vi "Get Visible Chart Data.vi"(7 "Selection Chart":refnum<vi>, 9 "error in (no error)":errorcluster) -> (1 "error out":errorcluster, 2 "waveform out":waveform(dbl), 4 "Y Length":i32)   [LabVIEW 2012]
uses:
  <vilib>/Waveform/WDTOps.llb/WDT Append Waveforms DBL.vi
  <vilib>/Waveform/WDTOps.llb/WDT Get Waveform Subset DBL.vi
panel:
  out "Time":dbl
  out "Portion":dbl
  out "size(s)":i32
  out "t0":timestamp
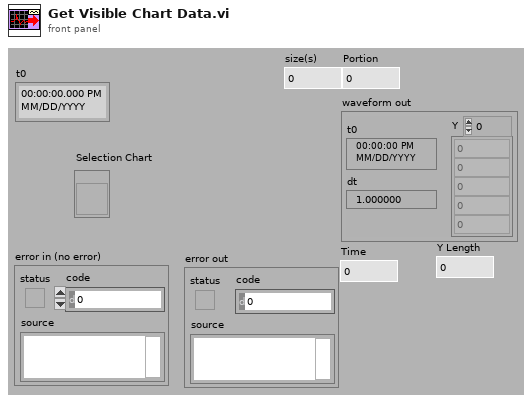
[diagram p1: front panel]
types:
  T1 = typedef "LVRangeTypeDef.ctl" = cluster{"Minimum":dbl, "Maximum":dbl, "Increment":dbl, "Minor Increment":dbl, "Start":dbl}
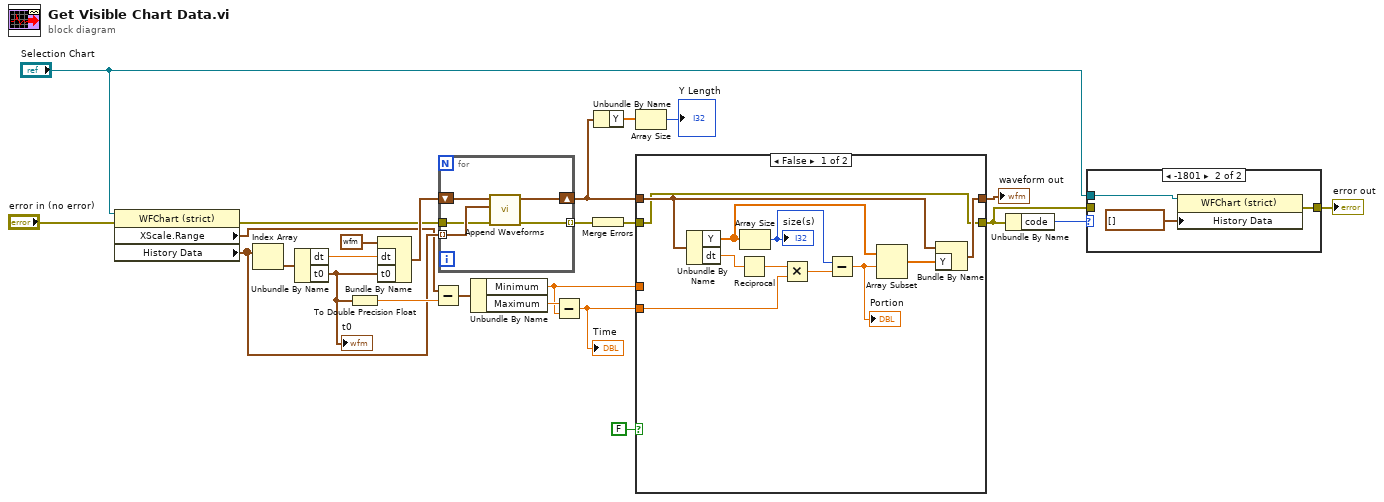
[diagram p0: block diagram]
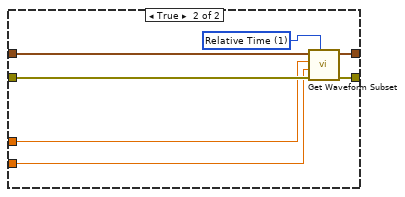
[diagram p2: hidden frame]
diagram:
  n1 = property class="WFChart (strict)"(reference="Selection Chart", error in="error in (no error)") -> (error out=w18:errorcluster, "XScale.Range"=w3:T1, "History Data"=w7:waveform(dbl)[])  [unwired: 1 out]
  n2 = Index Array(array=w7) -> (element=w6:waveform(dbl))  [unwired: 1 in]
  n3 = Unbundle By Name(w6) -> ("dt"=w20:dbl, "t0"=w17:timestamp)
  "t0" <- w17
  n4 = To Double Precision Float(number=w17) -> (double precision float=w15:dbl)
  n5 = Bundle By Name(cluster=waveform(dbl) {"t0"=timestamp(0 s since 1904-01-01), "dt"=2.267573696145e-05, "Y"=[]} ("waveform out"), "dt"=w20, "t0"=w17) -> (w22:waveform(dbl))
  n6 = Subtract(x=w3, y=w15) -> (x-y=w16:T1)
  n7 = for {
    tunnel: w7 -> [w29] mode=indexing
    shift-right: [w30] -> w5
    shift-left: w22 -> [w28]
    tunnel: w18 -> [w27]
    tunnel: [w26] -> w23 mode=indexing
    n8 = call-poly <vilib>:"Append Waveforms.vi"("error in (no error)"=w27, "waveform B"=w29, "waveform A"=w28) -> ("error out"=w26:errorcluster, "waveform out"=w30:waveform(dbl))  [unwired: 7 in]
  }
  n9 = Unbundle By Name(w16) -> ("Minimum"=w4:dbl, "Maximum"=w21:dbl)
  n10 = Subtract(x=w21, y=w4) -> (x-y=w2:dbl)
  "Time" <- w2
  n11 = Merge Errors(w23) -> (w24:errorcluster)
  n12 = Unbundle By Name(w5) -> ("Y"=w9:dbl[])
  n13 = Array Size(array=w9) -> (size(s)=→"Y Length":i32)
  n14 = case shown="False" FALSE {
    tunnel: w24 -> [w31 w48]
    tunnel: [w31 w46] -> w12
    tunnel: [w32 w45] -> w10
    tunnel: w5 -> [w35 w44]
    tunnel: w4 -> [_ w43]
    tunnel: w2 -> [w40 w42]
    frame False {
      n15 = Unbundle By Name(w35) -> ("Y"=w36:dbl[], "dt"=w38:dbl)
      n16 = Reciprocal(x=w38) -> (1/x=w37:dbl)
      n17 = Array Size(array=w36) -> (size(s)=w41:i32)
      "size(s)" <- w41
      n18 = Multiply(x=w37, y=w40) -> (x*y=w39:dbl)
      n19 = Subtract(x=w41, y=w39) -> (x-y=w33:dbl)
      "Portion" <- w33
      n20 = Array Subset(array=w36, index=w33) -> (w34:dbl[])  [unwired: 1 in]
      n21 = Bundle By Name(cluster=w35, "Y"=w34) -> (w32:waveform(dbl))
    }
    frame True {
      w47 = u16 1 items=["Samples", "Relative Time"] ("start/duration format")
      n22 = call-poly <vilib>:"Get Waveform Subset.vi"("start/duration format"=w47, "error in (no error)"=w48, "duration"=w42, "start samples/time"=w43, "waveform in"=w44) -> ("error out"=w46:errorcluster, "waveform out"=w45:waveform(dbl))  [unwired: 1 in, 2 out]
    }
  }
  "waveform out" <- w10
  n23 = Unbundle By Name(w12) -> ("code"=w14:i32)
  n24 = case shown="-1801" w14 {
    tunnel: "Selection Chart" -> [_ w51]
    tunnel: w12 -> [w49 _]
    tunnel: [w49 w50] -> w11
    frame 0, Default {
    }
    frame -1801 {
      n25 = property class="WFChart (strict)"(reference=w51, "History Data"=waveform(dbl)[] []) -> (error out=w50:errorcluster)  [unwired: 1 in, 1 out]
    }
  }
  "error out" <- w11
